vi "test channel create.vi"() -> (0 "dirs":T1[][](array[typedef]), 1 "types":T2[][](array[typedef]), 2 "names":string[][](array[string]), 3 "chans":refnum<class "TBM channel.lvclass">[][](array[class]), 4 "classification ok":bool, 5 "names ok":bool, 7 "types ok":bool)   [LabVIEW 2013, in "TBM Tests.lvlib"]
uses:
  TBM Tests.lvlib
  <vilib>/NI/Tag Bus/tag/Data Type.ctl
  channel/TBM channel.lvclass
  channel/channel classification.ctl
  <vilib>/NI/Tag Bus/tag/tag descriptor.lvclass/tag descriptor.ctl
  channel/TBM channel.lvclass/TBM channel.ctl
  <vilib>/NI/Tag Bus/tag/read tag name.vi
  <vilib>/NI/Tag Bus/tag/read data type.vi
  channel/Read channel classification.vi
  <vilib>/NI/Tag Bus/tag/tag descriptor.lvclass
  <vilib>/NI/Configuration Framework/serializable configuration/NISE_CEF_serializable configuration.lvclass
panel:
  out "uuid":string
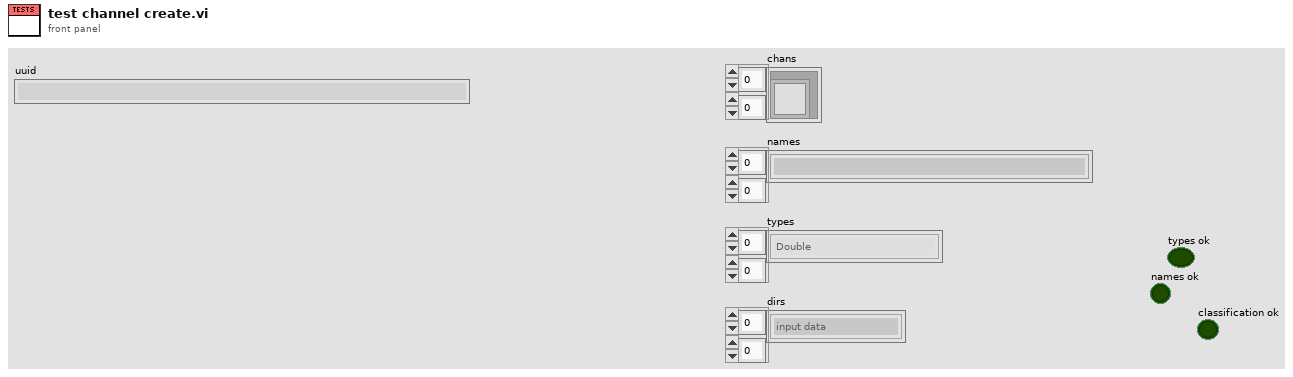
[diagram p1: front panel]
types:
  T1 = typedef "TBM channel.lvclass/channel classification.ctl" = enum16{"input data", "output data", "processing parameter", "processing result"}
  T2 = typedef "tag bus.lvlib/tag descriptor.lvclass/Data Type.ctl" = enum16{"Double", "Single", "I64", "I32", "I16", "I8", "U64", "U32", "U16", "U8", "Boolean", "String", "Array of Double", "Array of Single", "Array of I64", "Array of I32", "Array of I16", "Array of I8", "Array of U64", "Array of U32", "Array of U16", "Array of U8", "Array of Boolean", "Array of String"}
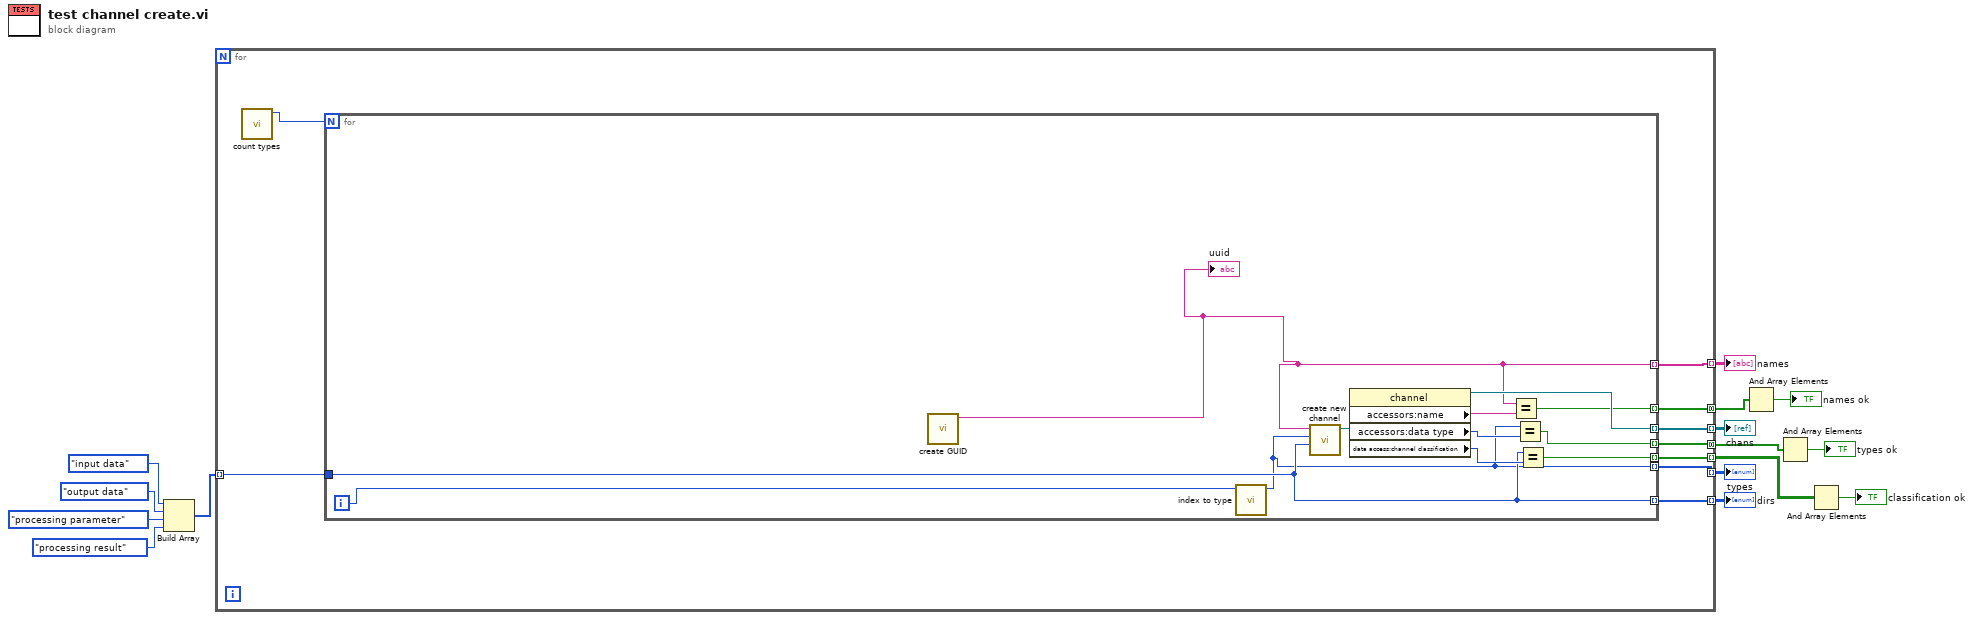
[diagram p0: block diagram]
diagram:
  n1 = Build Array(channel_classification."input data" ("channel classification"), channel_classification."output data" ("channel classification"), channel_classification."processing parameter" ("channel classification"), channel_classification."processing result" ("channel classification")) -> (w11:T1[])
  n2 = for {
    tunnel: w11 -> [w23] mode=indexing
    tunnel: [w22] -> w10 mode=indexing
    tunnel: [w21] -> w9 mode=indexing
    tunnel: [w20] -> w8 mode=indexing
    tunnel: [w19] -> w7 mode=indexing
    tunnel: [w18] -> w3 mode=concatenating
    tunnel: [w17] -> w6 mode=concatenating
    tunnel: [w16] -> w1 mode=indexing
    n3 = call <vilib>:"count types.vi"() -> ("type count"=w24:i32)  [unwired: 11 in]
    n4 = for {
      N: w24 -> [_]
      tunnel: w23 -> [w28]
      tunnel: [w25] -> w22 mode=indexing
      tunnel: [w26] -> w21 mode=indexing
      tunnel: [w34] -> w20 mode=indexing
      tunnel: [w28] -> w19 mode=indexing
      tunnel: [w30] -> w18 mode=indexing
      tunnel: [w29] -> w17 mode=indexing
      tunnel: [w27] -> w16 mode=indexing
      i -> [w36]
      n5 = call <vilib>:"create GUID.vi"() -> ("uuid"=w25:string)  [unwired: 10 in, 1 out]
      "uuid" <- w25
      n6 = call <vilib>:"index to type.vi"("I32"=w36) -> ("type"=w26:T2)  [unwired: 10 in]
      n7 = call "create new channel.vi"("channel classification"=w28, "data type"=w26, "channel name"=w25) -> ("channel"=w35:refnum<class "TBM channel.lvclass">)  [unwired: 8 in]
      n8 = property class="channel"(reference=w35) -> (reference out=w34:refnum<class "TBM channel.lvclass">, "accessors:name"=w31:string, "accessors:data type"=w32:T2, "data access:channel classification"=w33:T1)  [unwired: 1 in, 1 out]
      n9 = Equal?(x=w25, y=w31) -> (x = y?=w30:bool)
      n10 = Equal?(x=w26, y=w32) -> (x = y?=w29:bool)
      n11 = Equal?(x=w28, y=w33) -> (x = y?=w27:bool)
    }
  }
  "names" <- w10
  "types" <- w9
  "chans" <- w8
  "dirs" <- w7
  n12 = And Array Elements(Boolean array=w3) -> (logical AND=→"names ok":bool)
  n13 = And Array Elements(Boolean array=w6) -> (logical AND=→"types ok":bool)
  n14 = And Array Elements(Boolean array=w1) -> (logical AND=→"classification ok":bool)
